vi "sv_Shift and Low Pass Filter (N Ch Array) with IC.vi"(0 "input signals":dbl[][](array[numeric]), 1 "reset? (F)":bool, 5 "t0":dbl, 7 "center":dbl, 9 "decimation factor":i32, 11 "error in (no error)":errorcluster, 12 "initial conditions":T2 {"filter settings"."filters"."coefficients" format="%.2f"}, 13 "new dt":dbl) -> (4 "enveloped signals":dbl[][](array[numeric]), 6 "t0 out":dbl, 14 "final conditions":T2 {"filter settings"."filters"."coefficients" format="%.2f"}, 15 "error out":errorcluster)   [LabVIEW 2017, in "SoundVib_FaultAnalysis.lvlib"]
uses:
  <vilib>/addons/Sound and Vibration/Order Analysis/Fault Analysis/SoundVib_FaultAnalysis.lvlib
  <vilib>/addons/_NISVFA/_Shared subVIs/Controls/OAT Decimation Filter.ctl
  <vilib>/addons/Sound and Vibration/Order Analysis/Resample Order Tracking/SubVIs/OAT Frequency Shift (Mixer).vi
  <vilib>/addons/Sound and Vibration/Order Analysis/Resample Order Tracking/SubVIs/oa_Decimation with CIC and Compensation Filter.vi
  <vilib>/addons/Sound and Vibration/Order Analysis/Fault Analysis/SubVIs/oa_Demodulation Initial States (1 Channel).vi
  <vilib>/addons/Sound and Vibration/Order Analysis/Adv Resampling/OAT Single Stage Decimation with IC.vi
  <vilib>/addons/Sound and Vibration/Order Analysis/Resample Order Tracking/SubVIs/OAT CIC Decimation.vi
  <vilib>/addons/Sound and Vibration/Order Analysis/Resample Order Tracking/SubVIs/oa_Interpolate Zeros Between Samples.vi
  <vilib>/addons/Sound and Vibration/Order Analysis/Resample Order Tracking/SubVIs/oa_Calculate Delay of CIC Decimation Interpolation Filter.vi
  <vilib>/addons/Sound and Vibration/Order Analysis/Resample Order Tracking/SubVIs/oa_Create CIC Compensation Filter.vi
  <vilib>/addons/Sound and Vibration/Order Analysis/Resample Order Tracking/SubVIs/oa_Create CIC LP Truncation Filter.vi
  <vilib>/addons/Sound and Vibration/Order Analysis/Resample Order Tracking/SoundVib_Resampling.lvlib
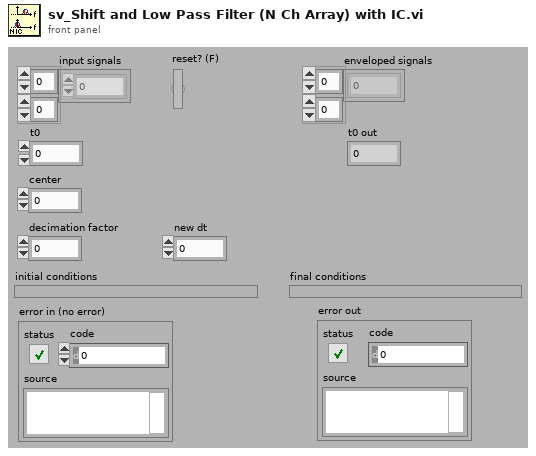
[diagram p1: front panel]
types:
  T1 = typedef "OAT Decimation Filter.ctl" = cluster{"coefficients":dbl[], "factor":i32}
  T2 = cluster{"filter settings":cluster{"CIC Settings":cluster{"Numeric":i32, i32, i32}, "filters":T1[], "delay":i32, "interpolation factor":i32}, "filter states":cluster{"t0":dbl, "phase":dbl, "real filter state":cluster{cluster{dbl[]}, cluster{dbl[]}[]}, "imaginary filter state":cluster{cluster{dbl[]}, cluster{dbl[]}[]}, "delay":i32}[], "reset pending":bool}
  T3 = cluster{"t0":dbl, "phase":dbl, "real filter state":cluster{cluster{dbl[]}, cluster{dbl[]}[]}, "imaginary filter state":cluster{cluster{dbl[]}, cluster{dbl[]}[]}, "delay":i32}[]
  T4 = cluster{"t0":dbl, "phase":dbl, "real filter state":cluster{cluster{dbl[]}, cluster{dbl[]}[]}, "imaginary filter state":cluster{cluster{dbl[]}, cluster{dbl[]}[]}, "delay":i32}
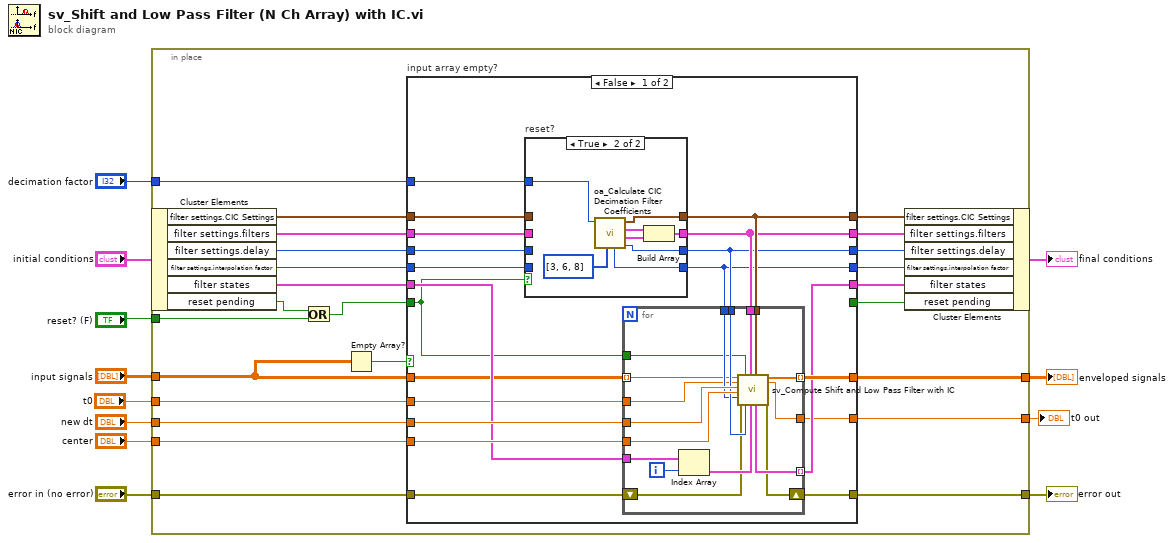
[diagram p0: block diagram]
diagram:
  n1 = in-place {
    in-place-border: "input signals" -> [w17]
    in-place-border: "decimation factor" -> [w36]
    in-place-border: "center" -> [w35]
    in-place-border: "new dt" -> [w34]
    in-place-border: "reset? (F)" -> [w21]
    in-place-border: [w33] -> w7
    in-place-border: "error in (no error)" -> [w16]
    in-place-border: [w15] -> w3
    in-place-border: [w14] -> w2
    in-place-border: "t0" -> [w13]
    n2 = in-place-cluster #1("initial conditions") -> ("filter settings.CIC Settings"=w30:cluster{"Numeric":i32, i32, i32}, "filter settings.filters"=w29:T1[], "filter settings.delay"=w28:i32, "filter settings.interpolation factor"=w27:i32, "filter states"=w32:T3, "reset pending"=w22:bool)
    n3 = Or(x=w22, y=w21) -> (x .or. y?=w20:bool)
    n4 = Empty Array?(array=w17) -> (empty?=w19:bool)
    n5 = case "input array empty?" shown="False" w19 {
      tunnel: w36 -> [w56 _]
      tunnel: w35 -> [w55 _]
      tunnel: w34 -> [w54 _]
      tunnel: [w53 w88] -> w33
      tunnel: w32 -> [w52 w89]
      tunnel: [w51 w89] -> w31
      tunnel: w30 -> [w50 w93]
      tunnel: w29 -> [w49 w92]
      tunnel: w28 -> [w48 w91]
      tunnel: w27 -> [w47 w90]
      tunnel: [w46 w93] -> w26
      tunnel: [w45 w92] -> w25
      tunnel: [w44 w91] -> w24
      tunnel: [w43 w90] -> w23
      tunnel: w20 -> [w42 w94]
      tunnel: [_ w94] -> w18
      tunnel: w17 -> [w41 w88]
      tunnel: w16 -> [w40 w87]
      tunnel: [w39 w87] -> w15
      tunnel: [w38 w86] -> w14
      tunnel: w13 -> [w37 w86]
      frame False {
        n6 = case "reset?" shown="True" w42 {
          tunnel: [w77 w85] -> w46
          tunnel: [w76 w82] -> w45
          tunnel: [w74 w81] -> w43
          tunnel: [w75 w80] -> w44
          tunnel: w56 -> [_ w79]
          tunnel: w50 -> [w77 _]
          tunnel: w49 -> [w76 _]
          tunnel: w48 -> [w75 _]
          tunnel: w47 -> [w74 _]
          frame False {
          }
          frame True {
            n7 = call <vilib>:"oa_Calculate CIC Decimation Filter Coefficients.vi"("CIC stages"=i32[] [3, 6, 8], "decimation/interpolation factor"=w79) -> ("delay"=w80:i32, "lp filter settings"=w83:T1, "compensation filter settings"=w84:T1, "CIC Settings"=w85:cluster{"Numeric":i32, i32, i32}, "interpolation factor"=w81:i32)  [unwired: 5 in]
            n8 = Build Array(w84, w83) -> (w82:T1[])
          }
        }
        n9 = for {
          tunnel: w55 -> [w73]
          tunnel: w54 -> [w72]
          tunnel: [w71] -> w53 mode=indexing
          tunnel: w52 -> [w65]
          tunnel: [w70] -> w51 mode=indexing
          tunnel: w46 -> [w59]
          tunnel: w45 -> [w60]
          tunnel: w44 -> [w69]
          tunnel: w43 -> [w68]
          tunnel: w42 -> [w67]
          tunnel: w41 -> [w66] mode=indexing
          shift-right: [w61] -> w39
          shift-left: w40 -> [w62]
          tunnel: [w58] -> w38
          tunnel: w37 -> [w57]
          i -> [w64]
          n10 = Index Array(array=w65, index=w64) -> (element=w63:T4)
          n11 = call <vilib>:"sv_Compute Shift and Low Pass Filter with IC.vi"("input signal"=w66, "t0"=w57, "new dt"=w72, "center"=w73, "interpolation factor"=w68, "error in (no error)"=w62, "reset? (F)"=w67, "delay"=w69, "filters"=w60, "initial conditions"=w63, "CIC settings"=w59) -> ("final conditions"=w70:T4, "enveloped signal"=w71:dbl[], "t0 out"=w58:dbl, "error out"=w61:errorcluster)  [unwired: 5 in]
        }
      }
      frame True {
      }
    }
    n12 = in-place-cluster #1("filter settings.CIC Settings"=w26, "filter settings.filters"=w25, "filter settings.delay"=w24, "filter settings.interpolation factor"=w23, "filter states"=w31, "reset pending"=w18) -> (→"final conditions":T2)
  }
  "enveloped signals" <- w7
  "error out" <- w3
  "t0 out" <- w2
